vi "HXGetMapID.vi"(0 "input":i32, 1 "output":i32, 2 "direction":enum16{"Input", "Output"}(ring), 3 "OldTerm":i32, 4 "Node type":T1(ring), 5 "Boolean":bool) -> (14 "Input":i32, 16 "Output":i32, 18 "MapID":i32)   [LabVIEW 2017]
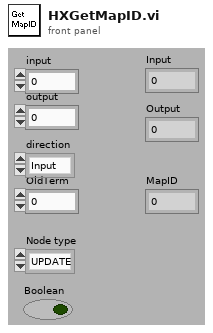
[diagram p1: front panel]
types:
  T1 = enum16{"UPDATE", "READ", "QUERY", "CREATE CHILD", "CREATE", "CONNECT", "DISCONNECT"}
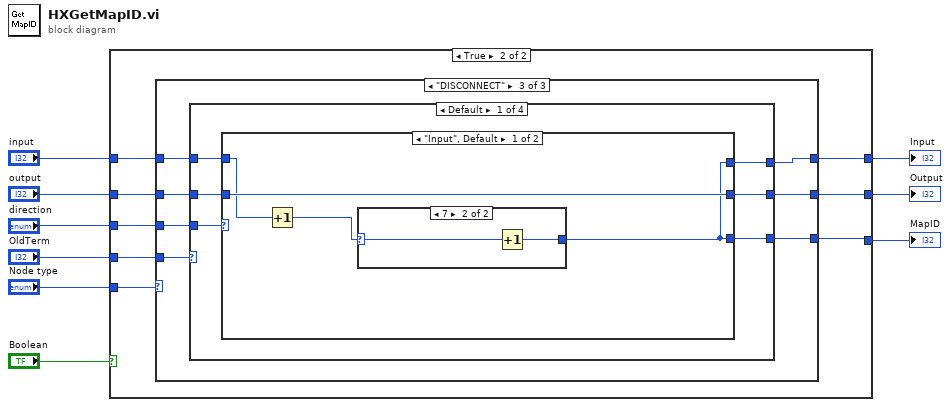
[diagram p0: block diagram]
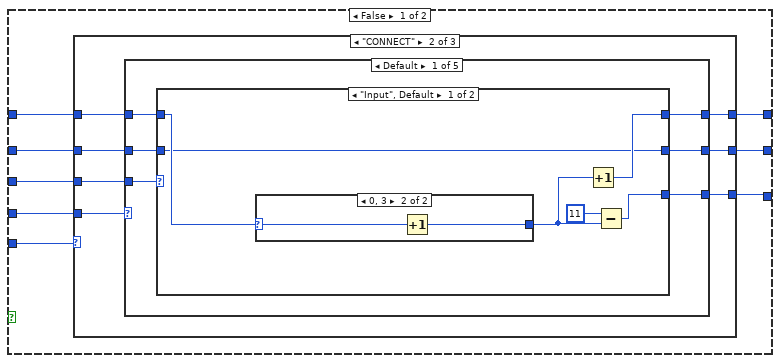
[diagram p2: hidden frame]
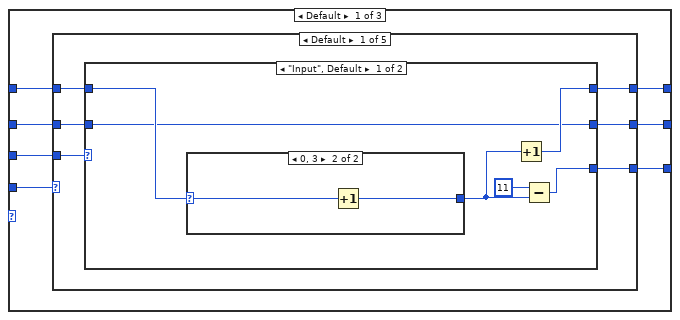
[diagram p3: hidden frame]
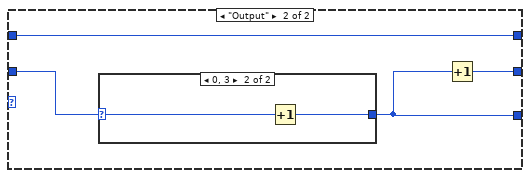
[diagram p5: hidden frame]
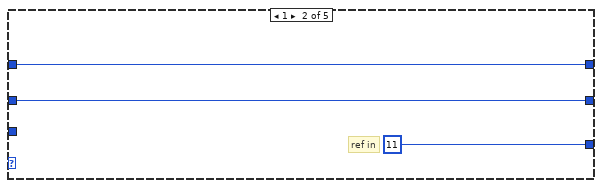
[diagram p7: hidden frame]
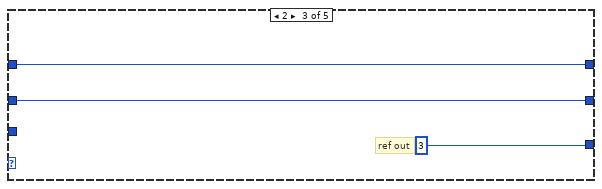
[diagram p8: hidden frame]
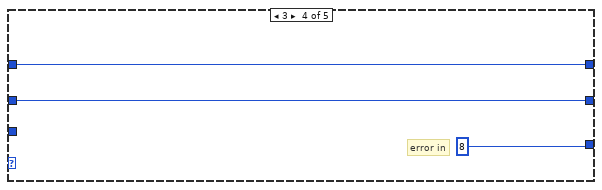
[diagram p9: hidden frame]
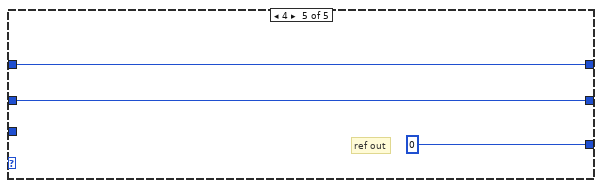
[diagram p10: hidden frame]
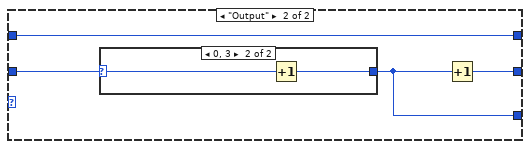
[diagram p12: hidden frame]
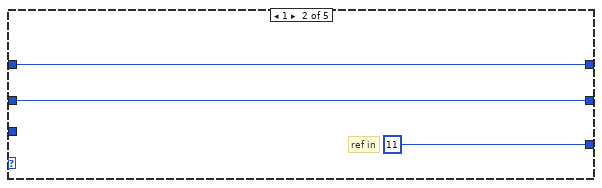
[diagram p14: hidden frame]
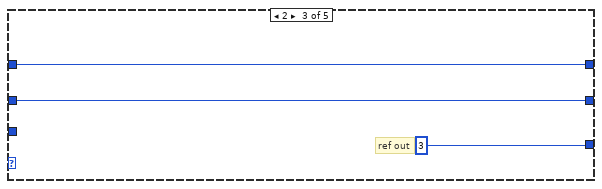
[diagram p15: hidden frame]
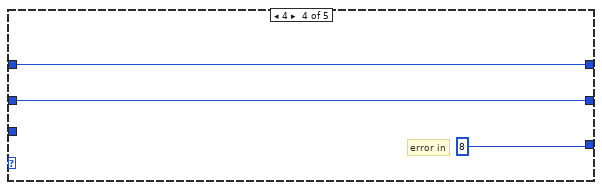
[diagram p16: hidden frame]
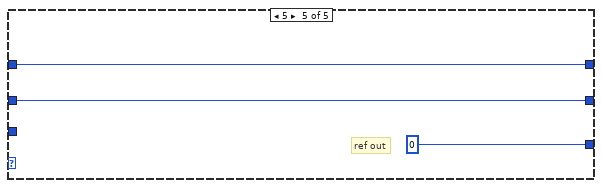
[diagram p17: hidden frame]
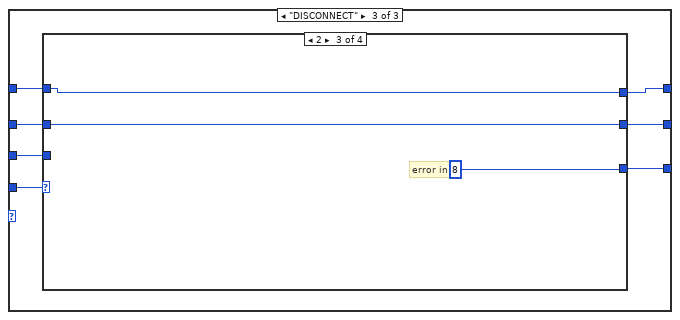
[diagram p18: hidden frame]
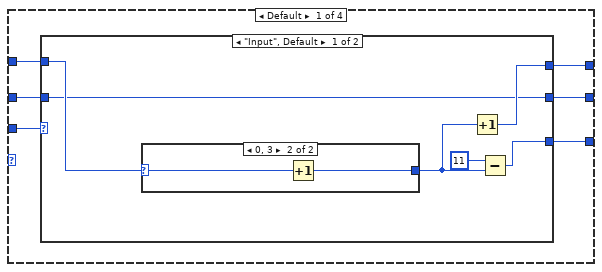
[diagram p19: hidden frame]
diagram:
  n1 = case shown="True" "Boolean" {
    tunnel: "Node type" -> [w17 w141]
    tunnel: "OldTerm" -> [w16 w142]
    tunnel: [w15 w138] -> w7
    tunnel: "input" -> [w14 w145]
    tunnel: "output" -> [w13 w144]
    tunnel: "direction" -> [w12 w143]
    tunnel: [w11 w139] -> w3
    tunnel: [w10 w140] -> w2
    frame False {
      n2 = case shown="\"CONNECT\"" w17 {
        tunnel: w16 -> [w24 w65 w103]
        tunnel: [w23 w59 w100] -> w15
        tunnel: w14 -> [w22 w62 w106]
        tunnel: w13 -> [w21 w63 w105]
        tunnel: w12 -> [w20 w64 w104]
        tunnel: [w19 w60 w101] -> w11
        tunnel: [w18 w61 w102] -> w10
        frame Default {
          n3 = case shown="Default" w24 {
            tunnel: [w28 11 3 8 0] -> w23
            tunnel: w22 -> [w26 w48 w51 w54 w57]
            tunnel: w21 -> [w29 w47 w50 w53 w56]
            tunnel: w20 -> [w30 _ _ _ _]
            tunnel: [w27 w47 w50 w53 w56] -> w19
            tunnel: [w25 w48 w51 w54 w57] -> w18
            frame Default {
              n4 = case shown="\"Input\", Default" w30 {
                tunnel: w29 -> [w31 w43]
                tunnel: [w33 w42] -> w28
                tunnel: [w31 w41] -> w27
                tunnel: w26 -> [w36 w40]
                tunnel: [w32 w40] -> w25
                frame "Input", Default {
                  n5 = case shown="0, 3" w36 {
                    selector: w36 -> [w37 w39]
                    tunnel: [w37 w38] -> w35
                    frame Default {
                    }
                    frame 0, 3 {
                      n6 = Increment(x=w39) -> (x+1=w38:i32)
                    }
                  }
                  n7 = Increment(x=w35) -> (x+1=w32:i32)
                  n8 = Subtract(x=11, y=w35) -> (x-y=w33:i32)
                }
                frame "Output" {
                  n9 = case shown="0, 3" w43 {
                    selector: w43 -> [w44 w46]
                    tunnel: [w44 w45] -> w42
                    frame Default {
                    }
                    frame 0, 3 {
                      n10 = Increment(x=w46) -> (x+1=w45:i32)
                    }
                  }
                  n11 = Increment(x=w42) -> (x+1=w41:i32)
                }
              }
            }
            frame 1 {
              # "ref in"
            }
            frame 2 {
              # "ref out"
            }
            frame 3 {
              # "error in"
            }
            frame 4 {
              # "ref out"
            }
          }
        }
        frame "CONNECT" {
          n12 = case shown="Default" w65 {
            tunnel: [w69 11 3 8 0] -> w59
            tunnel: w62 -> [w67 w89 w92 w95 w98]
            tunnel: w63 -> [w70 w88 w91 w94 w97]
            tunnel: w64 -> [w71 _ _ _ _]
            tunnel: [w68 w88 w91 w94 w97] -> w60
            tunnel: [w66 w89 w92 w95 w98] -> w61
            frame Default {
              n13 = case shown="\"Input\", Default" w71 {
                tunnel: w70 -> [w72 w84]
                tunnel: [w74 w83] -> w69
                tunnel: [w72 w82] -> w68
                tunnel: w67 -> [w77 w81]
                tunnel: [w73 w81] -> w66
                frame "Input", Default {
                  n14 = case shown="0, 3" w77 {
                    selector: w77 -> [w78 w80]
                    tunnel: [w78 w79] -> w76
                    frame Default {
                    }
                    frame 0, 3 {
                      n15 = Increment(x=w80) -> (x+1=w79:i32)
                    }
                  }
                  n16 = Increment(x=w76) -> (x+1=w73:i32)
                  n17 = Subtract(x=11, y=w76) -> (x-y=w74:i32)
                }
                frame "Output" {
                  n18 = case shown="0, 3" w84 {
                    selector: w84 -> [w85 w87]
                    tunnel: [w85 w86] -> w83
                    frame Default {
                    }
                    frame 0, 3 {
                      n19 = Increment(x=w87) -> (x+1=w86:i32)
                    }
                  }
                  n20 = Increment(x=w83) -> (x+1=w82:i32)
                }
              }
            }
            frame 1 {
              # "ref in"
            }
            frame 2 {
              # "ref out"
            }
            frame 4 {
              # "error in"
            }
            frame 5 {
              # "ref out"
            }
          }
        }
        frame "DISCONNECT" {
          n21 = case shown="2" w103 {
            tunnel: [w110 11 8 0] -> w100
            tunnel: w106 -> [w108 w130 w133 w136]
            tunnel: w105 -> [w111 w129 w132 w135]
            tunnel: w104 -> [w112 _ _ _]
            tunnel: [w109 w129 w132 w135] -> w101
            tunnel: [w107 w130 w133 w136] -> w102
            frame Default {
              n22 = case shown="\"Input\", Default" w112 {
                tunnel: w111 -> [w113 w125]
                tunnel: [w115 w124] -> w110
                tunnel: [w113 w123] -> w109
                tunnel: w108 -> [w118 w122]
                tunnel: [w114 w122] -> w107
                frame "Input", Default {
                  n23 = case shown="0, 3" w118 {
                    selector: w118 -> [w119 w121]
                    tunnel: [w119 w120] -> w117
                    frame Default {
                    }
                    frame 0, 3 {
                      n24 = Increment(x=w121) -> (x+1=w120:i32)
                    }
                  }
                  n25 = Increment(x=w117) -> (x+1=w114:i32)
                  n26 = Subtract(x=11, y=w117) -> (x-y=w115:i32)
                }
                frame "Output" {
                  n27 = case shown="0" w125 {
                    selector: w125 -> [w126 w128]
                    tunnel: [w126 w127] -> w124
                    frame Default {
                    }
                    frame 0 {
                      n28 = Increment(x=w128) -> (x+1=w127:i32)
                    }
                  }
                  n29 = Increment(x=w124) -> (x+1=w123:i32)
                }
              }
            }
            frame 1 {
              # "ref in"
            }
            frame 2 {
              # "error in"
            }
            frame 3 {
              # "error out"
            }
          }
        }
      }
    }
    frame True {
      n30 = case shown="\"DISCONNECT\"" w141 {
        tunnel: w142 -> [w152 w194 w232]
        tunnel: [w151 w188 w229] -> w138
        tunnel: w145 -> [w150 w191 w235]
        tunnel: w144 -> [w149 w192 w234]
        tunnel: w143 -> [w148 w193 w233]
        tunnel: [w147 w189 w230] -> w139
        tunnel: [w146 w190 w231] -> w140
        frame Default {
          n31 = case shown="Default" w152 {
            selector: w152 -> [w153 _ _ _ _]
            tunnel: [w157 0 20 7 27] -> w151
            tunnel: w150 -> [w155 w177 w180 w183 w186]
            tunnel: w149 -> [w158 w176 w179 w182 w185]
            tunnel: w148 -> [w159 _ _ _ _]
            tunnel: [w156 w176 w179 w182 w185] -> w147
            tunnel: [w154 w177 w180 w183 w186] -> w146
            frame Default {
              n32 = case shown="\"Input\", Default" w159 {
                tunnel: w158 -> [w163 w169]
                tunnel: [w160 w170] -> w157
                tunnel: [w163 w167] -> w156
                tunnel: w155 -> [w162 w172]
                tunnel: [w160 w172] -> w154
                tunnel: w153 -> [_ _]
                frame "Input", Default {
                  n33 = Increment(x=w162) -> (x+1=w161:i32)
                  n34 = case shown="Default" w161 {
                    selector: w161 -> [w164 w166]
                    tunnel: [w164 w165] -> w160
                    frame Default {
                    }
                    frame 7 {
                      n35 = Increment(x=w166) -> (x+1=w165:i32)
                    }
                  }
                }
                frame "Output" {
                  n36 = Increment(x=w169) -> (x+1=w168:i32)
                  n37 = case shown="7" w168 {
                    selector: w168 -> [w173 w175]
                    tunnel: [w173 w174] -> w167
                    frame Default {
                    }
                    frame 7 {
                      n38 = Increment(x=w175) -> (x+1=w174:i32)
                    }
                  }
                  n39 = Subtract(x=27, y=w167) -> (x-y=w170:i32)
                }
              }
            }
            frame 1 {
              # "ref in"
            }
            frame 2 {
              # "ref out"
            }
            frame 3 {
              # "error in"
            }
            frame 4 {
              # "ref out"
            }
          }
        }
        frame "CONNECT" {
          n40 = case shown="Default" w194 {
            tunnel: [w198 0 20 7 27] -> w188
            tunnel: w191 -> [w196 w218 w221 w224 w227]
            tunnel: w192 -> [w199 w217 w220 w223 w226]
            tunnel: w193 -> [w200 _ _ _ _]
            tunnel: [w197 w217 w220 w223 w226] -> w189
            tunnel: [w195 w218 w221 w224 w227] -> w190
            frame Default {
              n41 = case shown="\"Input\", Default" w200 {
                tunnel: w199 -> [w204 w212]
                tunnel: [w201 w210] -> w198
                tunnel: [w204 w208] -> w197
                tunnel: w196 -> [w203 w213]
                tunnel: [w201 w213] -> w195
                frame "Input", Default {
                  n42 = Increment(x=w203) -> (x+1=w202:i32)
                  n43 = case shown="7" w202 {
                    selector: w202 -> [w205 w207]
                    tunnel: [w205 w206] -> w201
                    frame Default {
                    }
                    frame 7 {
                      n44 = Increment(x=w207) -> (x+1=w206:i32)
                    }
                  }
                }
                frame "Output" {
                  n45 = Increment(x=w212) -> (x+1=w209:i32)
                  n46 = case shown="7" w209 {
                    selector: w209 -> [w214 w216]
                    tunnel: [w214 w215] -> w208
                    frame Default {
                    }
                    frame 7 {
                      n47 = Increment(x=w216) -> (x+1=w215:i32)
                    }
                  }
                  n48 = Subtract(x=27, y=w208) -> (x-y=w210:i32)
                }
              }
            }
            frame 1 {
              # "ref in"
            }
            frame 2 {
              # "ref out"
            }
            frame 4 {
              # "error in"
            }
            frame 5 {
              # "ref out"
            }
          }
        }
        frame "DISCONNECT" {
          n49 = case shown="Default" w232 {
            tunnel: [w239 0 7 27] -> w229
            tunnel: w235 -> [w237 w259 w262 w265]
            tunnel: w234 -> [w240 w258 w261 w264]
            tunnel: w233 -> [w241 _ _ _]
            tunnel: [w238 w258 w261 w264] -> w230
            tunnel: [w236 w259 w262 w265] -> w231
            frame Default {
              n50 = case shown="\"Input\", Default" w241 {
                tunnel: w240 -> [w245 w254]
                tunnel: [w242 w251] -> w239
                tunnel: [w245 w249] -> w238
                tunnel: w237 -> [w244 w253]
                tunnel: [w242 w253] -> w236
                frame "Input", Default {
                  n51 = Increment(x=w244) -> (x+1=w243:i32)
                  n52 = case shown="7" w243 {
                    selector: w243 -> [w246 w248]
                    tunnel: [w246 w247] -> w242
                    frame Default {
                    }
                    frame 7 {
                      n53 = Increment(x=w248) -> (x+1=w247:i32)
                    }
                  }
                }
                frame "Output" {
                  n54 = Increment(x=w254) -> (x+1=w250:i32)
                  n55 = case shown="7" w250 {
                    selector: w250 -> [w255 w257]
                    tunnel: [w255 w256] -> w249
                    frame Default {
                    }
                    frame 7 {
                      n56 = Increment(x=w257) -> (x+1=w256:i32)
                    }
                  }
                  n57 = Subtract(x=27, y=w249) -> (x-y=w251:i32)
                }
              }
            }
            frame 1 {
              # "ref in"
            }
            frame 2 {
              # "error in"
            }
            frame 3 {
              # "error out"
            }
          }
        }
      }
    }
  }
  "MapID" <- w7
  "Output" <- w3
  "Input" <- w2
